vi "CreateHistogram.vi"(11 "image data":T2) -> (3 "Histogram Graph":cluster{"Axis":dbl[], "Histogram":i32[]}[](graph))   [LabVIEW 2017]
uses:
  <vilib>/picture/picture.llb/imagedata.ctl
  <vilib>/Analysis/NI_AALPro.lvlib
panel:
  out "Array":T1(array[cluster])
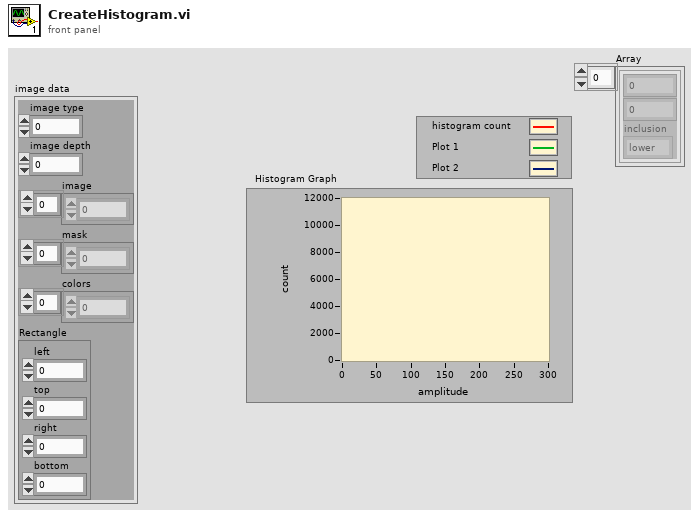
[diagram p1: front panel]
types:
  T1 = cluster{i32, i32, "inclusion":enum32{"lower", "upper", "both", "neither"}}[]
  T2 = typedef "imagedata.ctl" = cluster{"image type":i32, "image depth":i32, "image":u8[], "mask":u8[], "colors":u32[], "Rectangle":cluster{"left":i16, "top":i16, "right":i16, "bottom":i16}}
  T3 = cluster{i32, i32, "inclusion":enum32{"lower", "upper", "both", "neither"}}
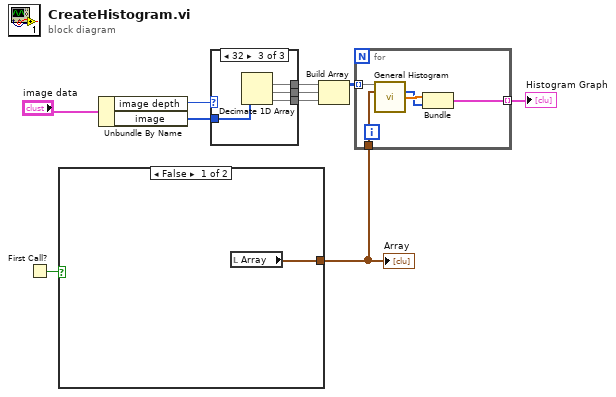
[diagram p0: block diagram]
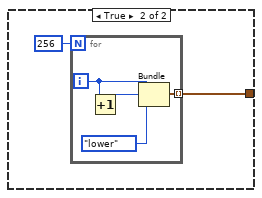
[diagram p2: hidden frame]
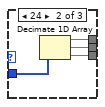
[diagram p4: hidden frame]
diagram:
  n1 = First Call?() -> (First Call?: T/F=w1:bool)
  n2 = case shown="False" w1 {
    tunnel: [w11 w12] -> w9
    frame False {
      n3 = local read "Array"() -> (w11:T1)
    }
    frame True {
      n4 = for {
        N: 256 -> [_]
        tunnel: [w14] -> w12 mode=indexing
        i -> [w16]
        n5 = Increment(x=w16) -> (x+1=w17:i32)
        n6 = Bundle(w16, w17, "inclusion"=enum32{"lower", "upper", "both", "neither"}."lower") -> (w14:T3)  [unwired: 1 out]
      }
    }
  }
  "Array" <- w9
  n7 = Unbundle By Name("image data") -> ("image depth"=w7:i32, "image"=w8:u8[])
  n8 = case shown="32" w7 {
    tunnel: [w18 w21 w25] -> w6
    tunnel: w8 -> [w18 w22 w26]
    tunnel: [w18 w20 w24] -> w5
    tunnel: [w18 w19 w23] -> w4
    frame Default {
    }
    frame 24 {
      n9 = Decimate 1D Array(w22) -> (w21:u8[], w20:u8[], w19:u8[])
    }
    frame 32 {
      n10 = Decimate 1D Array(w26) -> (w25:u8[], w24:u8[], w23:u8[])  [unwired: 1 out]
    }
  }
  n11 = Build Array(w6, w5, w4) -> (w3:u8[][])
  n12 = for {
    tunnel: w9 -> [w31]
    tunnel: w3 -> [w30] mode=indexing
    tunnel: [w27] -> w2 mode=indexing
    n13 = call <vilib>:"General Histogram.vi"("X"=w30, "Bins"=w31) -> ("Histogram"=w28:i32[], "Axis"=w29:dbl[])  [unwired: 4 in, 8 out]
    n14 = Bundle("Axis"=w29, "Histogram"=w28) -> (w27:cluster{"Axis":dbl[], "Histogram":i32[]})  [unwired: 1 in]
  }
  "Histogram Graph" <- w2
